vi "CalculateSampleRate.vi"(10 "Radio Buttons":T1=enum."Step 1") -> (3 "f":dbl format="%^#_6g")   [LabVIEW 2018]
uses:
  Controls/RadioButtons/FilterEnableRadio.ctl
panel:
  in  "EnableStep1":bool
  in  "Enable":T2
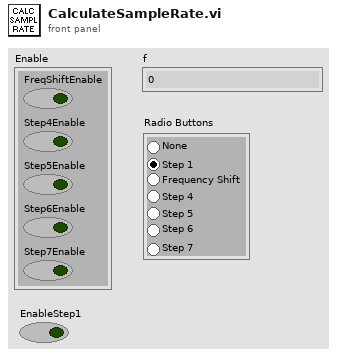
[diagram p1: front panel]
types:
  T1 = typedef "FilterEnableRadio.ctl" = enum32{"None", "Step 1", "Frequency Shift", "Step 4", "Step 5", "Step 6", "Step 7"}
  T2 = cluster{"FreqShiftEnable":bool, "Step4Enable":bool, "Step5Enable":bool, "Step6Enable":bool, "Step7Enable":bool}
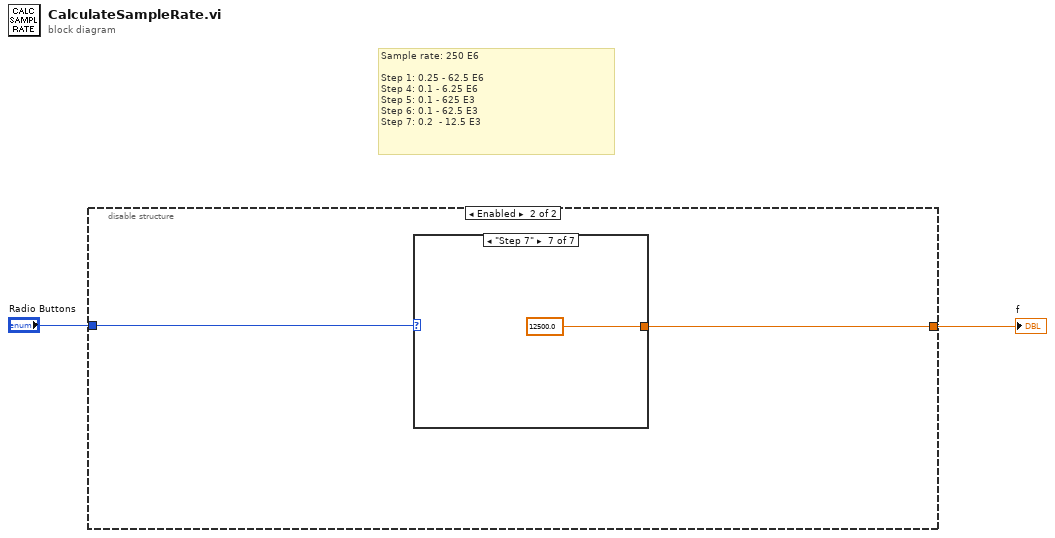
[diagram p0: block diagram]
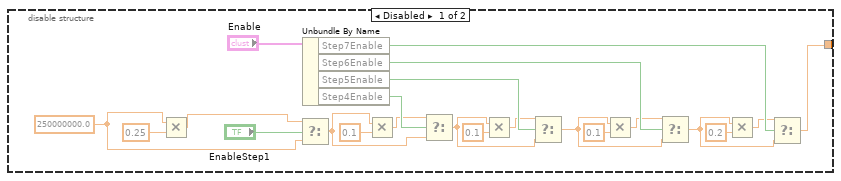
[diagram p2: hidden frame]
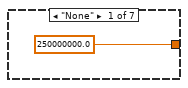
[diagram p3: hidden frame]
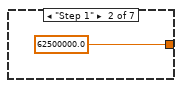
[diagram p4: hidden frame]
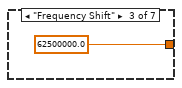
[diagram p5: hidden frame]
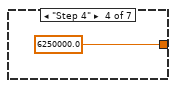
[diagram p6: hidden frame]
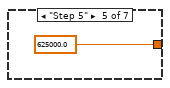
[diagram p7: hidden frame]
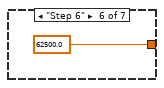
[diagram p8: hidden frame]
diagram:
  # "Sample rate: 250 E6\n\nStep 1: 0.25 - 62.5 E6\nStep 4: 0.1 - 6.25 E6\nStep 5: 0.1 - 625 E3\nStep 6: 0.1 - 62.5 E3\nStep 7: 0.2  - 12.5 E3"
  n1 = disable-structure shown="Enabled" {
    disable-tunnel: [w18 w25] -> w2
    disable-tunnel: "Radio Buttons" -> [_ w26]
    frame Disabled {
      w5 = 250000000.0 ("f")
      n2 = Multiply(x=w5, y=0.25) -> (x*y=w4:dbl)
      n3 = Select(t=w4, s="EnableStep1", f=w5) -> (s? t:f=w8:dbl)
      n4 = Unbundle By Name("Enable") -> ("Step7Enable"=w24:bool, "Step6Enable"=w23:bool, "Step5Enable"=w22:bool, "Step4Enable"=w21:bool)
      n5 = Multiply(x=w8, y=0.1) -> (x*y=w7:dbl)
      n6 = Select(t=w7, s=w21, f=w8) -> (s? t:f=w11:dbl)
      n7 = Multiply(x=w11, y=0.1) -> (x*y=w10:dbl)
      n8 = Select(t=w10, s=w22, f=w11) -> (s? t:f=w14:dbl)
      n9 = Multiply(x=w14, y=0.1) -> (x*y=w12:dbl)
      n10 = Select(t=w12, s=w23, f=w14) -> (s? t:f=w17:dbl)
      n11 = Multiply(x=w17, y=0.2) -> (x*y=w16:dbl)
      n12 = Select(t=w16, s=w24, f=w17) -> (s? t:f=w18:dbl)
    }
    frame Enabled {
      n13 = case shown="\"Step 7\"" w26 {
        tunnel: [250000000.0 ("f") 62500000.0 ("f") 62500000.0 ("f") 6250000.0 ("f") 625000.0 ("f") 62500.0 ("f") 12500.0 ("f")] -> w25
        frame "None" {
        }
        frame "Step 1" {
        }
        frame "Frequency Shift" {
        }
        frame "Step 4" {
        }
        frame "Step 5" {
        }
        frame "Step 6" {
        }
        frame "Step 7" {
        }
      }
    }
  }
  "f" <- w2
